vi "Configure Sample Mode.vi"(8 "error in (no error)":errorcluster, 9 "Number of Segments (2)":u16=2, 10 "Sample Mode (0: RealTime)":u16(ring) items=["RealTime", "RIS", "Sequence", "Roll", "WaveStream"], 11 "VISA resource name":refnum<visa-resource-name>) -> (0 "error out":errorcluster, 3 "VISA resource name out":refnum<visa-resource-name>)   [LabVIEW 2015, in "LeCroy Wave Series.lvlib"]
doc: "Controls the sample mode of the instrument. Choices are Real-time, Sequence, Roll, WaveStream, and RIS. Not all modes are available, depending upon the scope model, timebase setting, etc."
uses:
  <instrlib>/LeCroy Wave Series/LeCroy Wave Series.lvlib
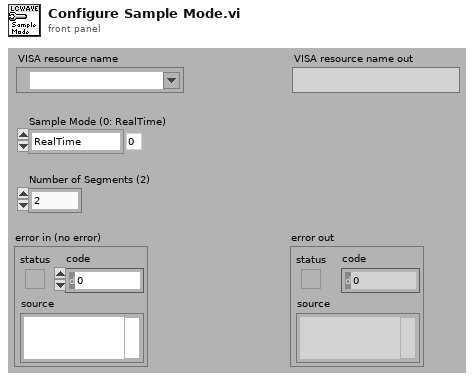
[diagram p1: front panel]
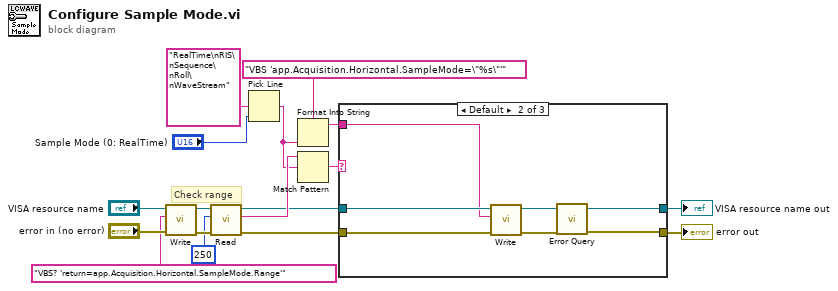
[diagram p0: block diagram]
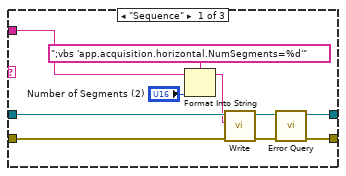
[diagram p2: hidden frame]
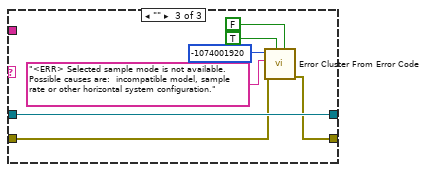
[diagram p3: hidden frame]
diagram:
  # "Check range"
  n1 = call <instrlib>:"Write.vi"("error in (no error)"="error in (no error)", "Write Buffer"="VBS? 'return=app.Acquisition.Horizontal.SampleMode.Range'" ("format string"), "VISA resource name"="VISA resource name") -> ("error out"=w15:errorcluster, "VISA resource name out"=w14:refnum<visa-resource-name>)  [unwired: 6 in, 1 out]
  n2 = call <instrlib>:"Read.vi"("error in (no error)"=w15, "Byte Count"=u32 250, "VISA resource name"=w14) -> ("error out"=w9:errorcluster, "Read Buffer"=w11:string, "VISA resource name out"=w10:refnum<visa-resource-name>)  [unwired: 5 in, 1 out]
  n3 = Pick Line(multi-line string="RealTime\nRIS\nSequence\nRoll\nWaveStream", line index="Sample Mode (0: RealTime)") -> (output string=w1:string)  [unwired: 1 in]
  n4 = Format Into String(format string="VBS 'app.Acquisition.Horizontal.SampleMode=\"%s\"'", w1) -> (resulting string=w8:string)  [unwired: 2 in, 1 out]
  n5 = Match Pattern(string=w11, regular expression=w1) -> (match substring=w6:string)  [unwired: 1 in, 3 out]
  n6 = case shown="Default" w6 {
    tunnel: w10 -> [w27 w34 w41]
    tunnel: w9 -> [w26 w33 w35]
    tunnel: w8 -> [w25 w32 _]
    tunnel: [w19 w29 w41] -> w4
    tunnel: [w20 w30 w36] -> w5
    frame "Sequence" {
      n7 = Format Into String(format string=";vbs 'app.acquisition.horizontal.NumSegments=%d'", initial string=w25, "Number of Segments (2)") -> (resulting string=w22:string)  [unwired: 1 in, 1 out]
      n8 = call <instrlib>:"Write.vi"("error in (no error)"=w26, "Write Buffer"=w22, "VISA resource name"=w27) -> ("error out"=w21:errorcluster, "VISA resource name out"=w18:refnum<visa-resource-name>)  [unwired: 6 in, 1 out]
      n9 = call <instrlib>:"Error Query.vi"("error in (no error)"=w21, "VISA resource name"=w18) -> ("error out"=w20:errorcluster, "VISA resource name out"=w19:refnum<visa-resource-name>)  [unwired: 6 in, 2 out]
    }
    frame Default {
      n10 = call <instrlib>:"Write.vi"("error in (no error)"=w33, "Write Buffer"=w32, "VISA resource name"=w34) -> ("error out"=w31:errorcluster, "VISA resource name out"=w28:refnum<visa-resource-name>)  [unwired: 6 in, 1 out]
      n11 = call <instrlib>:"Error Query.vi"("error in (no error)"=w31, "VISA resource name"=w28) -> ("error out"=w30:errorcluster, "VISA resource name out"=w29:refnum<visa-resource-name>)  [unwired: 6 in, 2 out]
    }
    frame "" {
      n12 = call <vilib>:"Error Cluster From Error Code.vi"("is warning? (False)"=FALSE, "show call chain? (False)"=TRUE, "error in (no error)"=w35, "error message (\"\")"="<ERR> Selected sample mode is not available. Possible causes are:  incompatible model, sample rate or other horizontal system configuration." ("source"), "error code (0)"=-1074001920 ("code")) -> ("error out"=w36:errorcluster)  [unwired: 4 in]
    }
  }
  "VISA resource name out" <- w4
  "error out" <- w5
